vi "GetClassDefiningMethod.vi"(8 "error in (no error)":errorcluster, 10 "MethodVI":refnum<vi>) -> (0 "error out":errorcluster, 2 "DefiningClass":string)   [LabVIEW 2013]
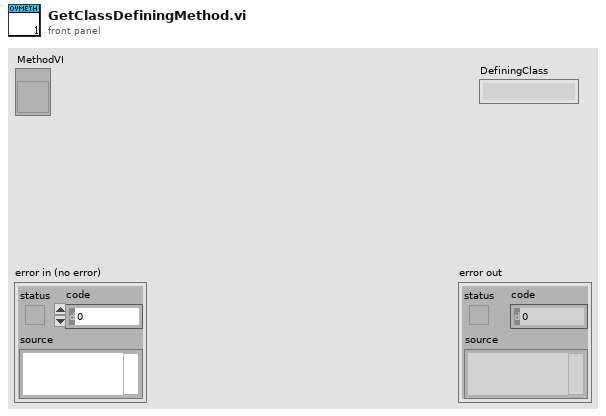
[diagram p1: front panel]
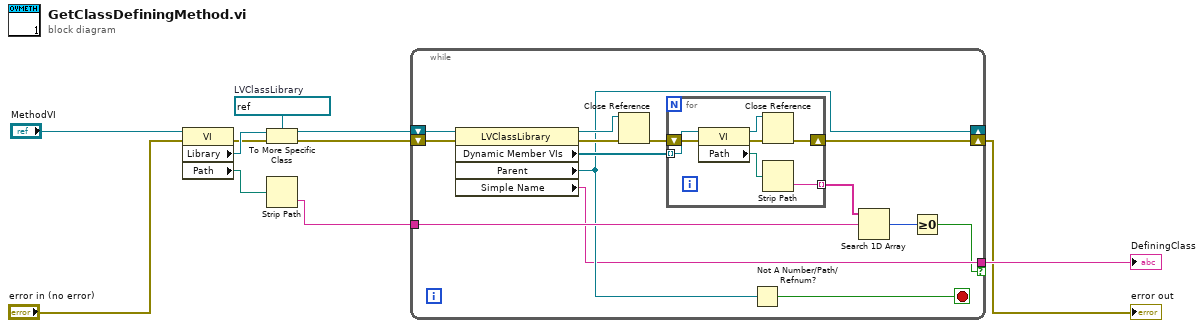
[diagram p0: block diagram]
diagram:
  w7 = refnum<vi> refnum  # LVClassLibrary
  n1 = property class="VI"(reference="MethodVI", error in="error in (no error)") -> (error out=w8:errorcluster, "Library"=w9:refnum<vi>, "Path"=w6:path)  [unwired: 1 out]
  n2 = To More Specific Class(target class=w7, reference=w9, error in=w8) -> (specific class reference=w3:refnum<vi>, error out=w4:errorcluster)
  n3 = Strip Path(path=w6) -> (name=w5:string)  [unwired: 1 out]
  n4 = while {
    tunnel: w5 -> [w25]
    shift-right: [w14] -> _
    shift-left: w3 -> [w18]
    shift-right: [w15] -> w1
    shift-left: w4 -> [w19]
    tunnel: [w13] -> w2 if=w12
    stop <- w17 stop-if-true
    n5 = property class="LVClassLibrary"(reference=w18, error in=w19) -> (reference out=w21:refnum<vi>, error out=w23:errorcluster, "Dynamic Member VIs"=w24:refnum<vi>[], "Parent"=w14:refnum<vi>, "Simple Name"=w13:string)
    n6 = Close Reference(reference=w21, error in (no error)=w23) -> (error out=w22:errorcluster)
    n7 = for {
      tunnel: w24 -> [w31] mode=indexing
      tunnel: [w29] -> w20 mode=indexing
      shift-right: [w27] -> w15
      shift-left: w22 -> [w32]
      n8 = property class="VI"(reference=w31, error in=w32) -> (reference out=w26:refnum<vi>, error out=w28:errorcluster, "Path"=w30:path)
      n9 = Close Reference(reference=w26, error in (no error)=w28) -> (error out=w27:errorcluster)
      n10 = Strip Path(path=w30) -> (name=w29:string)  [unwired: 1 out]
    }
    n11 = Not A Number/Path/Refnum?(number/path/refnum=w14) -> (NaN/Path/Refnum?=w17:bool)
    n12 = Search 1D Array(1D array=w20, element=w25) -> (index of element=w16:i32)  [unwired: 1 in]
    n13 = Greater Or Equal To 0?(x=w16) -> (x >= 0?=w12:bool)
  }
  "error out" <- w1
  "DefiningClass" <- w2
